vi "Get_Multical_Point.vi"(11 "Calib Fnames OUT":path[](array[path])) -> (2 "Cal Points":dbl[](array[numeric]), 3 "Ref Val":dbl)   [LabVIEW 2015]
doc: "Given an array of Calibration Filepaths, run the Calibration.vi to add a calibration data point to each file. Also, build an array containing the mean voltage for each of the FID channels included in the cal. Finally, dry-run Measurement.vi (not sure this is necessary)."
uses:
  ADAM Client/Sub VIs/ADAM Controls/Ch_description_ADAM.ctl
  ADAM Client/Sub VIs/ADAM Controls/Module_type_ADAM.ctl
  ADAM Client/Sub VIs/ADAM Controls/Function_ADAM.ctl
  ADAM Client/Sub VIs/ADAM Controls/Channel_State.ctl
  ADAM Client/Sub VIs/ADAM Controls/Calib_type_ADAM.ctl
  ADAM Client/Sub VIs/ADAM Controls/Address.ctl
  Anemometry Sub Vis/Controls/Setup.ctl
  Anemometry Sub Vis/Controls/Post_Process.ctl
  Anemometry Sub Vis/Controls/Save_Data.ctl
  Anemometry Sub Vis/Calibration/Calib_mode.ctl
  Anemometry Sub Vis/Controls/User_Specific_mode.ctl
  <vilib>/Analysis/baseanly.llb/Mean (DBL).vi
  Anemometry Sub Vis/Globals/Meas_global.vi
  <vilib>/Analysis/NI_AALBase.lvlib
panel:
  in  "Rig Gas Selector Ch":T1 {"Duty" format="%.0b"; "D" format="%#_5g"; "C" format="%#_5g"; "B" format="%#_5g"; "A" format="%#_5g"}
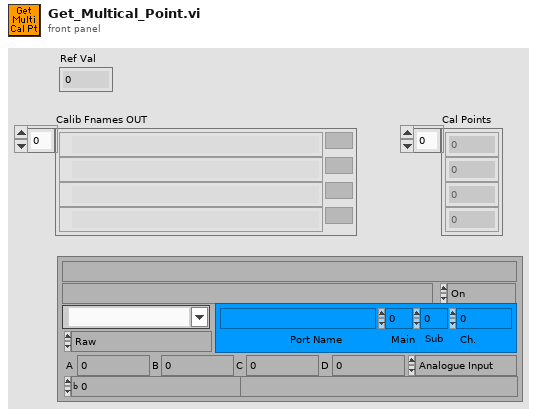
[diagram p1: front panel]
types:
  T1 = typedef "Ch_description_ADAM.ctl" = cluster{"Ch Name":string, "Type":T2, "Function":T3, "Ch State":T4, "Calibration type":T5, "A":dbl, "B":dbl, "C":dbl, "D":dbl, "Comments":string, "Address":T6, "String":string, "Duty":u16}
  T2 = typedef "Module_type_ADAM.ctl" = string
  T3 = typedef "Function_ADAM.ctl" = enum16{"Analogue Input", "Digital Input", "Event counter", "Event rate", "Analogue Output", "Digital Output", "Relay Output"}
  T4 = typedef "Channel_State.ctl" = enum16{"On", "Off", "Always On", "Always Off"}
  T5 = typedef "Calib_type_ADAM.ctl" = enum16{"Raw", "Bx + A", "Cx^2 + Bx + A", "Dx^3 + Cx^2 + Bx + A", "In Band", "Hi-Tec Q", "Hi-Tec M_dot", "Text"}
  T6 = typedef "Address.ctl" = cluster{"Main":i32, "Ch.":i32, "Sub":i32, "Port Name":string}
  T7 = typedef "Save_Data.ctl" = enum16{"Save No Data", "Save Data"}
  T8 = typedef "Post_Process.ctl" = enum16{"Take New Data", "Post Process Raw Data File"}
  T9 = typedef "Setup.ctl" = enum16{"Run Program", "Show Setup", "Save Current Setup", "Setup Front Panel"}
  T10 = typedef "User_Specific_mode.ctl" = enum16{"Check VI only", "Run VI"}
  T11 = typedef "Calib_mode.ctl" = enum16{"Show Setup", "Take a New Calibration Point", "Refit Curve", "Setup Front Panel"}
  T12 = typedef "Time_Trace_Cluster.ctl" = cluster{"Weighting":dbl[], "Time (s)":dbl[], "Voltage":dbl[], "Eng Values":dbl[]}
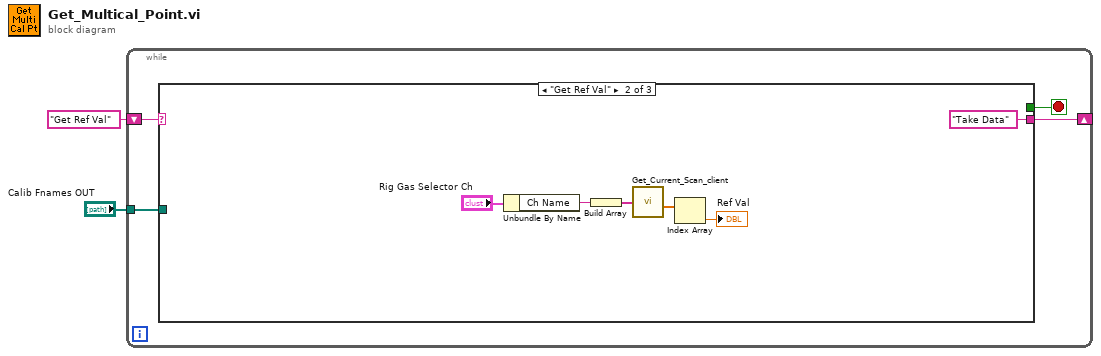
[diagram p0: block diagram]
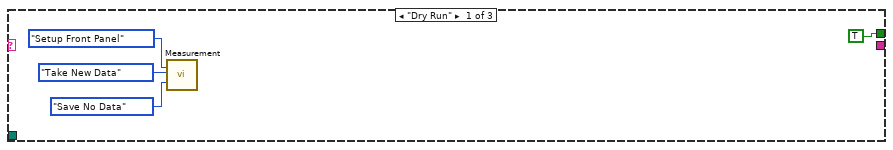
[diagram p2: hidden frame]
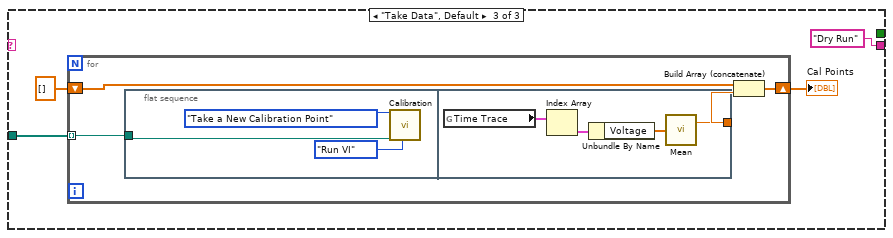
[diagram p3: hidden frame]
diagram:
  n1 = while {
    shift-right: [w5] -> _
    shift-left: "Get Ref Val" -> [w6]
    tunnel: "Calib Fnames OUT" -> [w3]
    stop <- w4 stop-if-true
    n2 = case shown="\"Get Ref Val\"" w6 {
      tunnel: [_ "Take Data" "Dry Run"] -> w5
      tunnel: [TRUE _ _] -> w4
      tunnel: w3 -> [_ _ w19]
      frame "Dry Run" {
        n3 = call "Measurement.vi"("setup"=Setup."Setup Front Panel", "Post Process"=Post_Process."Take New Data", "File"=Save_Data."Save No Data") -> ()  [unwired: 4 in, 13 out]
      }
      frame "Get Ref Val" {
        n4 = Unbundle By Name("Rig Gas Selector Ch") -> ("Ch Name"=w13:string)
        n5 = Build Array(w13) -> (w14:string[])
        n6 = call "Get_Current_Scan_client.vi"("ADAM Ch Names"=w14) -> ("Numerical Values"=w15:dbl[])  [unwired: 3 out]
        n7 = Index Array(array=w15) -> (element=→"Ref Val":dbl)  [unwired: 1 in]
      }
      frame "Take Data", Default {
        n8 = for {
          tunnel: w19 -> [w24] mode=indexing
          shift-right: [w22] -> w18
          shift-left: dbl[] [] -> [w21]
          n9 = flat-sequence {
            tunnel: w24 -> [w26]
            tunnel: [w28] -> w23
            frame #0 {
              n10 = call "Calibration.vi"("Mode"=Calib_mode."Take a New Calibration Point", "Calib file"=w26, "Simulate/Run"=User_Specific_mode."Run VI") -> ()  [unwired: 14 in, 3 out]
            }
            frame #1 {
              n11 = global read "Meas_global.vi" "Time Trace"() -> (w30:T12[])
              n12 = Index Array(array=w30) -> (element=w29:T12)  [unwired: 1 in]
              n13 = Unbundle By Name(w29) -> ("Voltage"=w31:dbl[])
              n14 = call-poly <vilib>:"Mean.vi"("X"=w31) -> ("mean"=w28:dbl)  [unwired: 1 out]
            }
          }
          n15 = Build Array (concatenate)(w21, w23) -> (w22:dbl[])
        }
        "Cal Points" <- w18
      }
    }
  }
